vi "MecaDrivePoseEst_SetVisionMeasurementStdDevs.vi"(10 "VisionMeasurementStdDevs":T1, 11 "in MecaDrivePoseEstimate":T2={"M_VisionContR"=[], "m_nominal_dT"=0.0, "m_PrevTime_Sec"=0.0, "m_GyroOffset"={"VALUE"=0.0, "COS"=1.0, "SIN"=0.0}, "m_PrevAngle"={"VALUE"=0.0, "COS"=1.0, "SIN"=0.0}, "m_Observer"={"m_P"=[], "m_xHat"=[], "States"=0, "Outputs"=0, "m_ContR"=[], "m_ContQ"=[], "m_SigmasF"=[], "m_dT_Sec"=0.0, "MERWE_SCALED_SIGMA_PTS"={"m_Wm"=[], "States"=0, "Alpha"=0.0, "m_Wc"=[], "Kappa"=0}, "meanFuncX"=refnum, "meanFuncY"=refnum, "residualFuncX"=refnum, "residualFuncY"=refnum, "addFuncX"=refnum, "addFuncXExtra"=variant, "residualFuncYExtra"=variant, "residualFuncXExtra"=variant, "MeanFuncYExtra"=variant, "MeanFuncXExtra"=variant, "Inputs"=0}, "m_kinematics"={"FrontLeft"={"X"=0.0, "Y"=0.0}, "FrontRight"={"X"=0.0, "Y"=0.0}, "RearLeft"={"X"=0.0, "Y"=0.0}, "RearRight"={"X"=0.0, "Y"=0.0}, "InverseKinematics"=[[0.0, 1.0, -1.0, 0.0], [0.0, 1.0, 1.0, 0.0], [0.0, 1.0, 1.0, 0.0], [0.0, 1.0, -1.0, 0.0]], "ForwardKinematics"=[[0.0, 1.0, -1.0, 0.0], [0.0, 1.0, 1.0, 0.0], [0.0, 1.0, 1.0, 0.0], [0.0, 1.0, -1.0, 0.0]], "PrevCoR"={"X"=0.0, "Y"=0.0}}, "Pose_Buffer"={"TimeStamps"=[], "Pose"=[], "Min_TimeStamp"=0.0, "Max_TimeStamp"=0.0, "ItemCount"=0, "MaxBufferTime"=0.0}} {"Pose_Buffer"."Pose"."ROTATION"."SIN" format="%13.4f"; "Pose_Buffer"."Pose"."ROTATION"."COS" format="%13.4f"; "Pose_Buffer"."Pose"."ROTATION"."VALUE" format="%13.4f"; "Pose_Buffer"."Pose"."TRANSLATION"."Y" format="%14.3f"; "Pose_Buffer"."Pose"."TRANSLATION"."X" format="%14.3f"; "m_kinematics"."PrevCoR"."Y" format="%14.3f"; "m_kinematics"."PrevCoR"."X" format="%14.3f"; "m_kinematics"."RearRight"."Y" format="%14.3f"; "m_kinematics"."RearRight"."X" format="%14.3f"; "m_kinematics"."RearLeft"."Y" format="%14.3f"; "m_kinematics"."RearLeft"."X" format="%14.3f"; "m_kinematics"."FrontRight"."Y" format="%14.3f"; "m_kinematics"."FrontRight"."X" format="%14.3f"; "m_kinematics"."FrontLeft"."Y" format="%14.3f"; "m_kinematics"."FrontLeft"."X" format="%14.3f"; "m_PrevAngle"."SIN" format="%13.4f"; "m_PrevAngle"."COS" format="%13.4f"; "m_PrevAngle"."VALUE" format="%13.4f"; "m_GyroOffset"."SIN" format="%13.4f"; "m_GyroOffset"."COS" format="%13.4f"; "m_GyroOffset"."VALUE" format="%13.4f"}) -> (0 "Size Coerced":bool, 3 "Out MecaDrivePoseEstimate":T2={"M_VisionContR"=[], "m_nominal_dT"=0.0, "m_PrevTime_Sec"=0.0, "m_GyroOffset"={"VALUE"=0.0, "COS"=1.0, "SIN"=0.0}, "m_PrevAngle"={"VALUE"=0.0, "COS"=1.0, "SIN"=0.0}, "m_Observer"={"m_P"=[], "m_xHat"=[], "States"=0, "Outputs"=0, "m_ContR"=[], "m_ContQ"=[], "m_SigmasF"=[], "m_dT_Sec"=0.0, "MERWE_SCALED_SIGMA_PTS"={"m_Wm"=[], "States"=0, "Alpha"=0.0, "m_Wc"=[], "Kappa"=0}, "meanFuncX"=refnum, "meanFuncY"=refnum, "residualFuncX"=refnum, "residualFuncY"=refnum, "addFuncX"=refnum, "addFuncXExtra"=variant, "residualFuncYExtra"=variant, "residualFuncXExtra"=variant, "MeanFuncYExtra"=variant, "MeanFuncXExtra"=variant, "Inputs"=0}, "m_kinematics"={"FrontLeft"={"X"=0.0, "Y"=0.0}, "FrontRight"={"X"=0.0, "Y"=0.0}, "RearLeft"={"X"=0.0, "Y"=0.0}, "RearRight"={"X"=0.0, "Y"=0.0}, "InverseKinematics"=[[0.0, 1.0, -1.0, 0.0], [0.0, 1.0, 1.0, 0.0], [0.0, 1.0, 1.0, 0.0], [0.0, 1.0, -1.0, 0.0]], "ForwardKinematics"=[[0.0, 1.0, -1.0, 0.0], [0.0, 1.0, 1.0, 0.0], [0.0, 1.0, 1.0, 0.0], [0.0, 1.0, -1.0, 0.0]], "PrevCoR"={"X"=0.0, "Y"=0.0}}, "Pose_Buffer"={"TimeStamps"=[], "Pose"=[], "Min_TimeStamp"=0.0, "Max_TimeStamp"=0.0, "ItemCount"=0, "MaxBufferTime"=0.0}} {"Pose_Buffer"."Pose"."ROTATION"."SIN" format="%13.4f"; "Pose_Buffer"."Pose"."ROTATION"."COS" format="%13.4f"; "Pose_Buffer"."Pose"."ROTATION"."VALUE" format="%13.4f"; "Pose_Buffer"."Pose"."TRANSLATION"."Y" format="%14.3f"; "Pose_Buffer"."Pose"."TRANSLATION"."X" format="%14.3f"; "m_kinematics"."PrevCoR"."Y" format="%14.3f"; "m_kinematics"."PrevCoR"."X" format="%14.3f"; "m_kinematics"."RearRight"."Y" format="%14.3f"; "m_kinematics"."RearRight"."X" format="%14.3f"; "m_kinematics"."RearLeft"."Y" format="%14.3f"; "m_kinematics"."RearLeft"."X" format="%14.3f"; "m_kinematics"."FrontRight"."Y" format="%14.3f"; "m_kinematics"."FrontRight"."X" format="%14.3f"; "m_kinematics"."FrontLeft"."Y" format="%14.3f"; "m_kinematics"."FrontLeft"."X" format="%14.3f"; "m_PrevAngle"."SIN" format="%13.4f"; "m_PrevAngle"."COS" format="%13.4f"; "m_PrevAngle"."VALUE" format="%13.4f"; "m_GyroOffset"."SIN" format="%13.4f"; "m_GyroOffset"."COS" format="%13.4f"; "m_GyroOffset"."VALUE" format="%13.4f"})   [LabVIEW 2019, in "Trajectory_Library.lvlib"]
doc: "Sets the pose estimator's trust of global measurements. This might be used to change trust in vision measurements after the autonomous period, or to change trust as distance to a vision target increases.\n \nInputs:\n - SwervePoseEst -- Data cluster containing SwervePoseEst data\n - visionMeasurementStdDevs -- Standard deviations of the vision measurements. Increase these\n numbers to trust global measurements from vision less. This matrix is in the form \n \n [x, y,theta]?, \n with units in meters and radians.\n \nOutputs:\n - outSwevePoseEst -- Updated data cluster \n - SizeCoereced -- If TRUE, an unexpected error occured. Execution may continue."
uses:
  Trajectory_Library.lvlib
  MECA_DRIVE_POSE_EST.ctl
  <vilib>/Analysis/Matrix/Datatypes/RealMatrix.ctl
  ROTATION2D.ctl
  UNSCENTED_KALMAN_FILTER.ctl
  MERWE_SCALED_SIGMA_PTS.ctl
  CALLBACK_FUNC_TYPE.ctl
  MECA_DRIVE_KINEMATICS.ctl
  TRANSLATION2D.ctl
  TIME_INTERPOLATABLE_POSE2D.ctl
  POSE2D.ctl
  MatBuilder_Create.vi
  MatrixHelper_CoerceSize.vi
  <vilib>/Analysis/Matrix/NI_Matrix.lvlib
panel:
  # "<3, 1>"
  # "<3, 3>"
  # "State Estimate <Statess,1>"
  # "<States, States>"
  # "<States, ?>"
  # "<Statess,  States>"
  # "<Outputs, Outputs>"
  # "<?, 1>"
  # "<?, 1>"
  # "<3, 3>"
  # "State Estimate <Statess,1>"
  # "<States, States>"
  # "<States, ?>"
  # "<Statess,  States>"
  # "<Outputs, Outputs>"
  # "<?, 1>"
  # "<?, 1>"
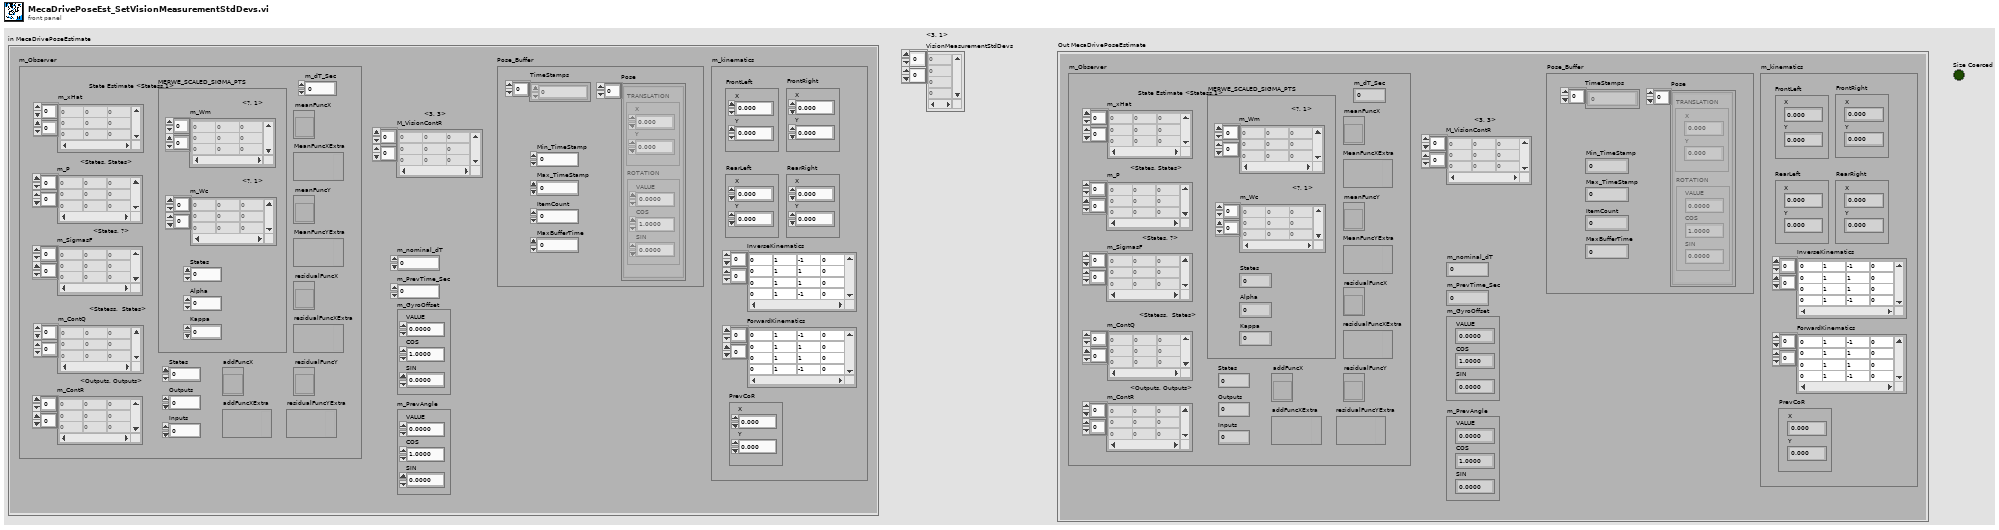
[diagram p1: front panel]
types:
  T1 = typedef "NI_Matrix.lvlib/RealMatrix.ctl" = dbl[][]
  T2 = typedef "Trajectory_Library.lvlib/MECA_DRIVE_POSE_EST.ctl" = cluster{"M_VisionContR":T1, "m_nominal_dT":dbl, "m_PrevTime_Sec":dbl, "m_GyroOffset":T3, "m_PrevAngle":T3, "m_Observer":T4, "m_kinematics":T7, "Pose_Buffer":T9}
  T3 = typedef "Trajectory_Library.lvlib/ROTATION2D.ctl" = cluster{"VALUE":dbl, "COS":dbl, "SIN":dbl}
  T4 = typedef "Trajectory_Library.lvlib/UNSCENTED_KALMAN_FILTER.ctl" = cluster{"m_P":T1, "m_xHat":T1, "States":i32, "Outputs":i32, "m_ContR":T1, "m_ContQ":T1, "m_SigmasF":T1, "m_dT_Sec":dbl, "MERWE_SCALED_SIGMA_PTS":T5, "meanFuncX":T6, "meanFuncY":T6, "residualFuncX":T6, "residualFuncY":T6, "addFuncX":T6, "addFuncXExtra":variant, "residualFuncYExtra":variant, "residualFuncXExtra":variant, "MeanFuncYExtra":variant, "MeanFuncXExtra":variant, "Inputs":i32}
  T5 = typedef "Trajectory_Library.lvlib/MERWE_SCALED_SIGMA_PTS.ctl" = cluster{"m_Wm":T1, "States":i32, "Alpha":dbl, "m_Wc":T1, "Kappa":i32}
  T6 = typedef "Trajectory_Library.lvlib/CALLBACK_FUNC_TYPE.ctl" = refnum<vi>
  T7 = typedef "Trajectory_Library.lvlib/MECA_DRIVE_KINEMATICS.ctl" = cluster{"FrontLeft":T8, "FrontRight":T8, "RearLeft":T8, "RearRight":T8, "InverseKinematics":T1, "ForwardKinematics":T1, "PrevCoR":T8}
  T8 = typedef "Trajectory_Library.lvlib/TRANSLATION2D.ctl" = cluster{"X":dbl, "Y":dbl}
  T9 = typedef "Trajectory_Library.lvlib/TIME_INTERPOLATABLE_POSE2D.ctl" = cluster{"TimeStamps":dbl[], "Pose":T10[], "Min_TimeStamp":dbl, "Max_TimeStamp":dbl, "ItemCount":i32, "MaxBufferTime":dbl}
  T10 = typedef "Trajectory_Library.lvlib/POSE2D.ctl" = cluster{"TRANSLATION":T8, "ROTATION":T3}
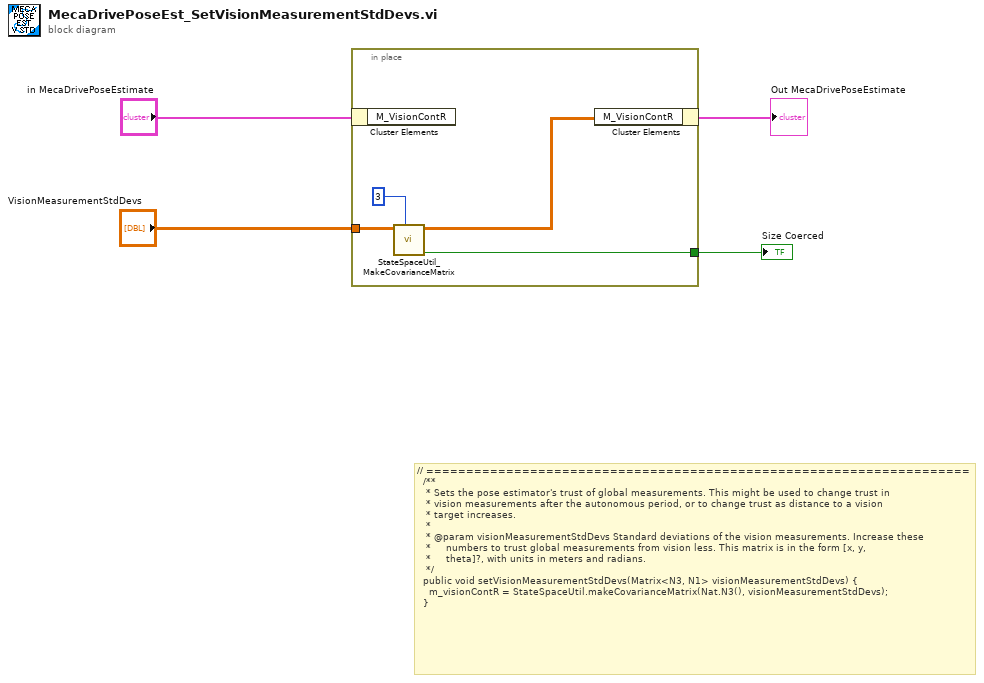
[diagram p0: block diagram]
diagram:
  # "// ====================================================================\n  /**\n   * Sets the pose estimator's trust of global measurements. This might be used to change trust in\n   * vision measurements after the autonomous period, or to change trust as distance to a vision\n   * target increases.\n   *\n   * @param visionMeasurementStdDevs Standard deviations of the vision measurements. Increase these\n   *     numbers to trust global measurements from vision less. This matrix is in the form [x, y,\n   *     theta]?, with units in meters and radians.\n   */\n  public void setVisionMeasurementStdDevs(Matrix<N3, N1> visionMeasurementStdDevs) {\n    m_visionContR = StateSpaceUtil.makeCovarianceMatrix(Nat.N3(), visionMeasurementStdDevs);\n  }"
  n1 = in-place {
    in-place-border: "VisionMeasurementStdDevs" -> [w8]
    in-place-border: [w5] -> w1
    n2 = in-place-cluster #1("in MecaDrivePoseEstimate") -> ()  [unwired: 1 out]
    n3 = call "StateSpaceUtil_MakeCovarianceMatrix.vi"("States"=3, "StdDevs"=w8) -> ("Size Coerced"=w5:bool, "Covariance Matrix"=w6:T1)  [unwired: 8 in]
    n4 = in-place-cluster #1("M_VisionContR"=w6) -> (→"Out MecaDrivePoseEstimate":T2)
  }
  "Size Coerced" <- w1
